vi "Test Helper Loop waiting for Stop.vi"(8 "error in (no error)":errorcluster, 11 "Helper Loop Test In":refnum<class "Helper Loop Test.lvclass">) -> (0 "error out":errorcluster, 3 "Helper Loop Test Out":refnum<class "Helper Loop Test.lvclass">)   [LabVIEW 2020, in "Helper Loop Test.lvclass"]
uses:
  Helper Loop Test.lvclass
  C:/Program Files (x86)/National Instruments/LabVIEW 2020/vi.lib/Asteme/LUnit/Test Case.lvclass
  Mock Process/Mock Process.lvclass
  C:/Users/anton/Documents/GitHub/Triarc-Framework/source/Framework/Process/Process.lvclass
  Framework/Process/Process.lvclass/Process.ctl
  <vilib>/Asteme/LUnit/Test Case.lvclass/Test Case.ctl
  <vilib>/Asteme/LUnit/LUnit Assertion Result.lvclass/LUnit Assertion Result.ctl
  Framework/Process/Public/Get Lifecycle State.vi
  Framework/Process/Private/SubVIs/Wait for finish.vi
  Framework/Process/Protected/Messaging/Enqueue Message.vi
  Framework/Process/Private/SubVIs/Set Lifecycle State.vi
  <vilib>/Asteme/LUnit/Palette/Fail.vi
  <vilib>/Asteme/LUnit/Palette/Pass.vi
  <vilib>/Asteme/LUnit/Set Assertion Type.vi
  <vilib>/Utility/error.llb/Clear Errors.vi
  <vilib>/Asteme/LUnit/Add test result.vi
  <vilib>/Asteme/LUnit/LUnit Write Passed.vi
  <vilib>/Asteme/LUnit/LUnit Get Test Case.vi
  <vilib>/Asteme/LUnit/LUnit Write Message.vi
  <vilib>/Asteme/LUnit/LUnit Write Description.vi
  <vilib>/Asteme/LUnit/LUnit Write Assertion Type.vi
  <vilib>/Asteme/LUnit/Read Test Case Name.vi
  <vilib>/Utility/error.llb/Error Cluster From Error Code.vi
  Support/Event Helpers/Dequeue Event Message.vi
  <vilib>/Asteme/LUnit/Assertion Result/LUnit Get Test Name.vi
  <vilib>/Asteme/LUnit/LUnit Assertion Result.lvclass
  Framework/Process/Process.lvclass
  <vilib>/Asteme/LUnit/Test Case.lvclass
  Support/Framework Test Support.lvlib
  Support/Event Helpers/Event Helpers.lvlib
panel:
  out "x >= y?":bool
  out "Current or Duration [ms] 2":u32
  out "Current or Duration [ms]":u32
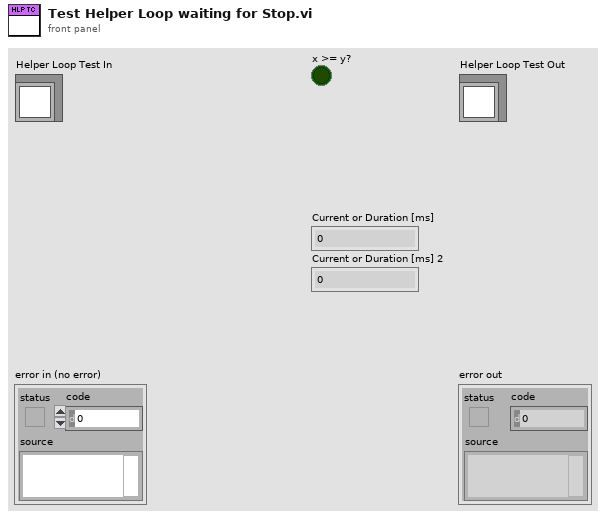
[diagram p1: front panel]
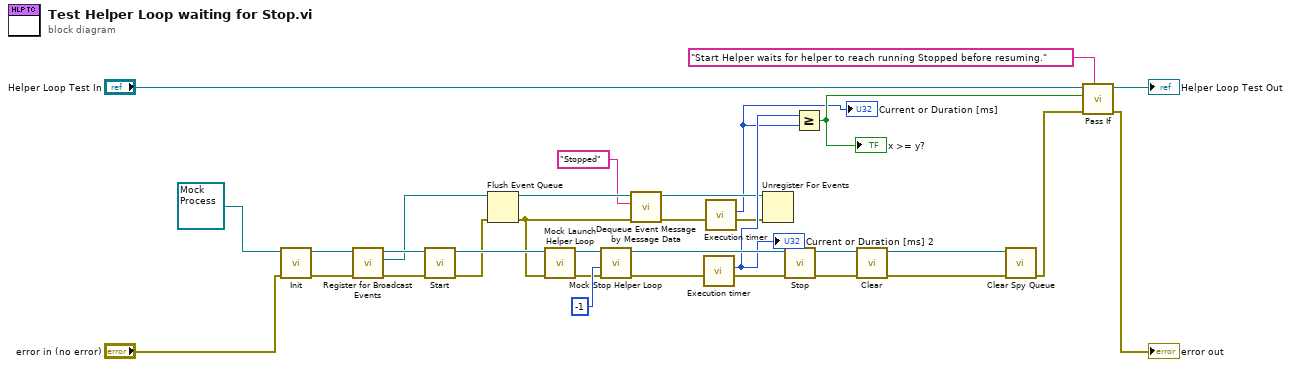
[diagram p0: block diagram]
diagram:
  n1 = call-dynamic "Init.vi"("error in (no error)"="error in (no error)", "Mock Process In"=refnum<class "Mock Process.lvclass"> refnum) -> ("error out"=w31:errorcluster, "Mock Process Out"=w32:refnum<class "Mock Process.lvclass">)  [unwired: 8 in]
  n2 = call-dynamic "Register for Broadcast Events.vi"("error in (no error)"=w31, "Process In"=w32) -> ("error out"=w29:errorcluster, "Event Registration Refnum"=w14:refnum<event-registration>, "Process Out"=w30:refnum<class "Mock Process.lvclass">)  [unwired: 7 in]
  n3 = call "Start.vi"("error in (no error)"=w29, "Process In"=w30) -> ("error out"=w12:errorcluster, "Process Out"=w28:refnum<class "Mock Process.lvclass">)  [unwired: 8 in]
  n4 = Flush Event Queue(0:w14, 3:w12) -> (8:w13:refnum<event-registration>, 11:w7:errorcluster)  [unwired: 4 in, 1 out]
  n5 = call "Mock Launch Helper Loop.vi"("error in (no error)"=w7, "Mock Process in"=w28) -> ("error out"=w4:errorcluster, "Mock Process out"=w27:refnum<class "Mock Process.lvclass">)  [unwired: 8 in]
  n6 = call "Mock Stop Helper Loop.vi"("error in (no error)"=w4, "timeout in ms (-1)"=-1, "Mock Process in"=w27) -> ("error out"=w3:errorcluster, "Mock Process out"=w26:refnum<class "Mock Process.lvclass">)  [unwired: 6 in, 1 out]
  n7 = call "Dequeue Event Message by Message Data.vi"("error in (no error)"=w7, "Message Data"="Stopped", "Event Registration Refnum"=w13) -> ("error out"=w11:errorcluster, "Event Registration Refnum Out"=w8:refnum<event-registration>)  [unwired: 4 in, 3 out]
  n8 = call "Execution timer.vi"("error in (no error)"=w3) -> ("error out"=w2:errorcluster, "Current or Duration [ms]"=w10:u32)  [unwired: 9 in]
  "Current or Duration [ms] 2" <- w10
  n9 = call "Execution timer.vi"("error in (no error)"=w11) -> ("error out"=w9:errorcluster, "Current or Duration [ms]"=w1:u32)  [unwired: 9 in]
  "Current or Duration [ms]" <- w1
  n10 = Unregister For Events(event registration refnum=w8, error in=w9) -> ()  [unwired: 1 out]
  n11 = call "Stop.vi"("error in (no error)"=w2, "Process In"=w26) -> ("error out"=w24:errorcluster, "Process Out"=w25:refnum<class "Mock Process.lvclass">)  [unwired: 7 in, 1 out]
  n12 = Greater Or Equal?(x=w10, y=w1) -> (x >= y?=w6:bool)
  "x >= y?" <- w6
  n13 = call-dynamic "Clear.vi"("error in (no error)"=w24, "Mock Process In"=w25) -> ("error out"=w22:errorcluster, "Mock Process Out"=w23:refnum<class "Mock Process.lvclass">)  [unwired: 8 in]
  n14 = call-dynamic "Clear Spy Queue.vi"("error in (no error)"=w22, "Mock Process In"=w23) -> ("error out"=w18:errorcluster)  [unwired: 8 in, 1 out]
  n15 = call <vilib>:"Pass If.vi"("Description"="Start Helper waits for helper to reach running Stopped before resuming.", "error in (no error)"=w18, "Pass?"=w6, "Test Case In"="Helper Loop Test In") -> ("error out"=→"error out":errorcluster, "Test Case Out"=→"Helper Loop Test Out":refnum<class "Helper Loop Test.lvclass">)  [unwired: 6 in]
